vi "ZCAN_InitCAN( CANET ).vi"(0 "设备类型":u32, 5 "device_hande":u32, 7 "CANindex":u32, 9 "ZCAN_InitCAN_setting_CANET":T1, 11 "error in (no error)":errorcluster caption="错误输入（无错误）") -> (8 "can_index_handle":u32, 15 "error out":errorcluster caption="错误输出")   [LabVIEW 2018]
doc: "用于设置CAN通道的初始化参数。\n\n适用的设备：CANET-TCP ,CANET-UDP"
uses:
  zlgcan_demo_CANFDNET_UDP/bin/zlgcan_wrap.dll
  data_type/ZCAN_InitCAN_setting_CANET.ctl
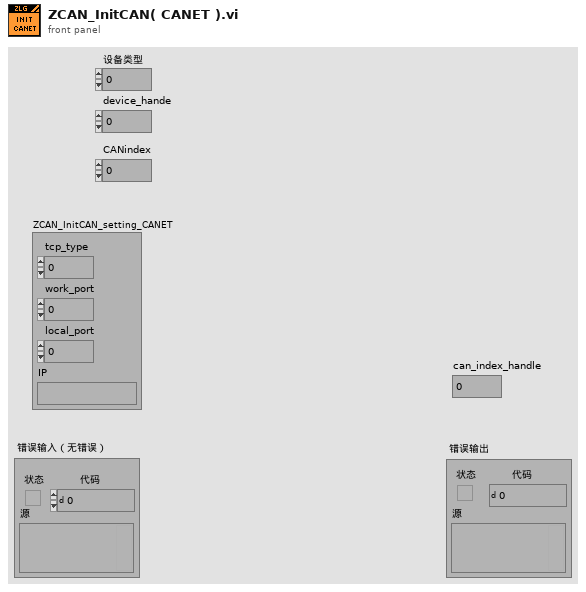
[diagram p1: front panel]
types:
  T1 = typedef "ZCAN_InitCAN_setting_CANET.ctl" = cluster{"tcp_type":u32, "work_port":u32, "local_port":u32, "IP":string}
  T2 = cluster{"can_type":u32, "can_type":u32, "can_type":u32, "can_type":u32, "can_type":u32, "can_type":u32, u8, u8, "pad":u16, "reserved":u32}
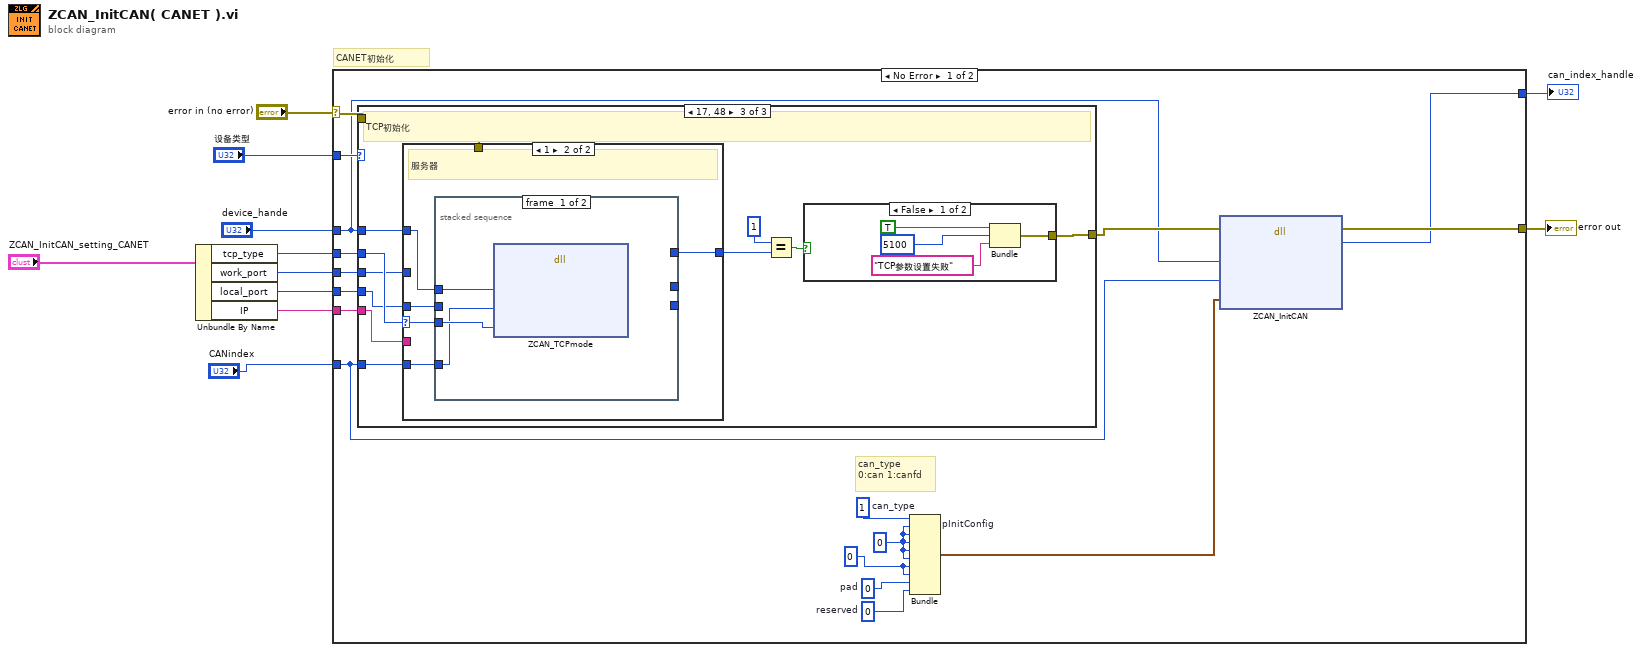
[diagram p0: block diagram]
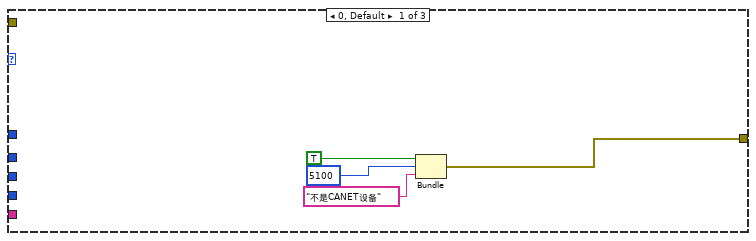
[diagram p2: hidden frame]
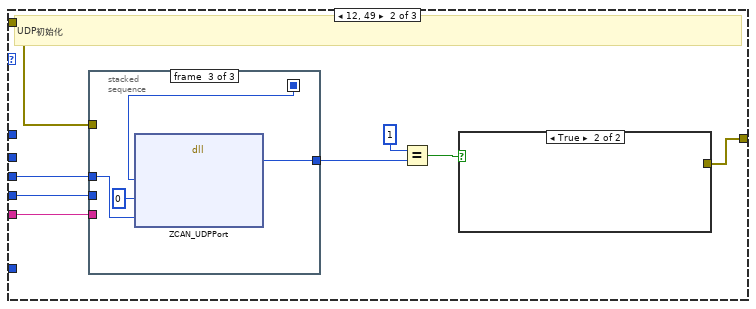
[diagram p3: hidden frame]
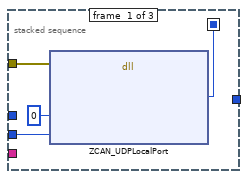
[diagram p4: hidden frame]
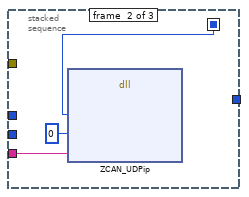
[diagram p5: hidden frame]
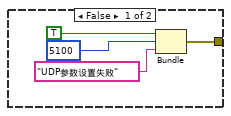
[diagram p6: hidden frame]
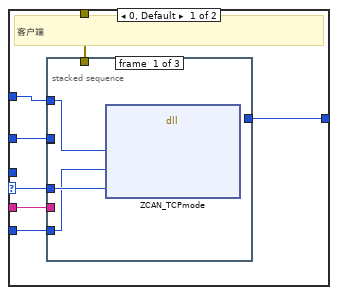
[diagram p7: hidden frame]
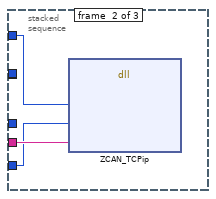
[diagram p8: hidden frame]
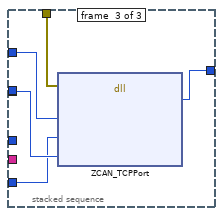
[diagram p9: hidden frame]
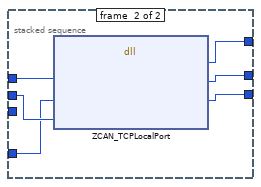
[diagram p10: hidden frame]
diagram:
  # "CANET初始化"
  n1 = Unbundle By Name("ZCAN_InitCAN_setting_CANET") -> ("tcp_type"=w9:u32, "work_port"=w7:u32, "local_port"=w6:u32, "IP"=w8:string)
  n2 = case shown="No Error" "error in (no error)" {
    selector: "error in (no error)" -> [w24 w104]
    tunnel: [w16 w104] -> w4
    tunnel: "设备类型" -> [w23 _]
    tunnel: "device_hande" -> [w14 w103]
    tunnel: w9 -> [w28 _]
    tunnel: w8 -> [w27 _]
    tunnel: w7 -> [w26 _]
    tunnel: w6 -> [w25 _]
    tunnel: [w13 w103] -> w5
    tunnel: "CANindex" -> [w12 _]
    frame No Error {
      w18 = u8 0
      w20 = u32 0  # reserved
      w21 = u16 0  # pad
      w19 = u32 0 ("can_type")
      w22 = u32 1  # can_type
      # "can_type\n0:can 1:canfd"
      n3 = case "条件结构" shown="17, 48" w23 {
        tunnel: [w29 w40 w58] -> w17
        tunnel: w14 -> [_ _ w63]
        tunnel: w28 -> [_ _ w62]
        tunnel: w27 -> [_ w38 w61]
        tunnel: w26 -> [_ w37 w60]
        tunnel: w25 -> [_ w39 w57]
        tunnel: w24 -> [_ w33 w59]
        tunnel: w12 -> [_ _ w56]
        frame 0, Default {
          n4 = Bundle("status"=TRUE, "code"=5100, "消息"="不是CANET设备") -> (w29:cluster{"status":bool, "code":i32, "消息":string})  [unwired: 1 in]
        }
        frame 12, 49 {
          # "UDP初始化"
          n5 = stacked-sequence {
            seq-local: [w41 _ _] -> [_ w45 w48]
            tunnel: w39 -> [w43 _ _]
            tunnel: w38 -> [_ w47 _]
            tunnel: w37 -> [_ _ w51]
            tunnel: [_ _ w49] -> w34
            tunnel: w33 -> [w42 _ _]
            frame #0 {
              n6 = dll-call lib="C:/Users/admin/Desktop/zlgcan_demo_CANFDNET_UDP/bin/zlgcan_wrap.dll" fn="ZCAN_UDPLocalPort"(error in=w42, "can_index"=u32 0, "local_port"=w43) -> ("hDev"=w41:u32)  [unwired: 6 in, 2 out]
            }
            frame #1 {
              n7 = dll-call lib="C:/Users/admin/Desktop/zlgcan_demo_CANFDNET_UDP/bin/zlgcan_wrap.dll" fn="ZCAN_UDPip"("device_handle"=w45, "can_index"=u32 0, "ip"=w47) -> ()  [unwired: 7 in, 2 out]
            }
            frame #2 {
              n8 = dll-call lib="C:/Users/admin/Desktop/zlgcan_demo_CANFDNET_UDP/bin/zlgcan_wrap.dll" fn="ZCAN_UDPPort"("hDev"=w48, "can_index"=u32 0, "work_port"=w51) -> ("return"=w49:u32)  [unwired: 6 in, 2 out]
            }
          }
          n9 = Equal?(x=1, y=w34) -> (x = y?=w35:bool)
          n10 = case shown="True" w35 {
            tunnel: [w52 _] -> w40
            frame False {
              n11 = Bundle("status"=TRUE, "code"=5100, "消息"="UDP参数设置失败") -> (w52:cluster{"status":bool, "code":i32, "消息":string})  [unwired: 1 in]
            }
            frame True {
            }
          }
        }
        frame 17, 48 {
          # "TCP初始化"
          n12 = case shown="1" w62 {
            selector: w62 -> [w73 w89]
            tunnel: [w72 w88] -> w65
            tunnel: w63 -> [w71 w87]
            tunnel: w61 -> [w70 _]
            tunnel: w60 -> [w69 _]
            tunnel: w59 -> [w68 _]
            tunnel: w57 -> [_ w86]
            tunnel: w56 -> [w67 w85]
            frame 0, Default {
              # "客户端"
              n13 = stacked-sequence {
                tunnel: w73 -> [w76 _ _]
                tunnel: [_ _ w84] -> w72
                tunnel: w71 -> [w75 w78 w83]
                tunnel: w70 -> [_ w79 _]
                tunnel: [_ _ w82] -> _
                tunnel: w69 -> [_ _ w82]
                tunnel: w68 -> [_ _ w81]
                tunnel: w67 -> [w74 w77 w80]
                frame #0 {
                  n14 = dll-call lib="C:/Users/admin/Desktop/zlgcan_demo_CANFDNET_UDP/bin/zlgcan_wrap.dll" fn="ZCAN_TCPmode"("hDev"=w75, "can_index"=w74, "tcp_type"=w76) -> ()  [unwired: 7 in, 2 out]
                }
                frame #1 {
                  n15 = dll-call lib="C:/Users/admin/Desktop/zlgcan_demo_CANFDNET_UDP/bin/zlgcan_wrap.dll" fn="ZCAN_TCPip"("device_handle"=w78, "can_index"=w77, "ip"=w79) -> ()  [unwired: 7 in, 2 out]
                }
                frame #2 {
                  n16 = dll-call lib="C:/Users/admin/Desktop/zlgcan_demo_CANFDNET_UDP/bin/zlgcan_wrap.dll" fn="ZCAN_TCPPort"(error in=w81, "hDev"=w83, "can_index"=w80, "work_port"=w82) -> ("return"=w84:u32)  [unwired: 5 in, 2 out]
                }
              }
            }
            frame 1 {
              # "服务器"
              n17 = stacked-sequence {
                tunnel: w89 -> [w92 _]
                tunnel: [_ w98] -> w88
                tunnel: [_ w97] -> _
                tunnel: [_ w96] -> _
                tunnel: w87 -> [w91 w94]
                tunnel: w86 -> [_ w95]
                tunnel: w85 -> [w90 w93]
                frame #0 {
                  n18 = dll-call lib="C:/Users/admin/Desktop/zlgcan_demo_CANFDNET_UDP/bin/zlgcan_wrap.dll" fn="ZCAN_TCPmode"("hDev"=w91, "can_index"=w90, "tcp_type"=w92) -> ()  [unwired: 7 in, 2 out]
                }
                frame #1 {
                  n19 = dll-call lib="C:/Users/admin/Desktop/zlgcan_demo_CANFDNET_UDP/bin/zlgcan_wrap.dll" fn="ZCAN_TCPLocalPort"("device_handle"=w94, "can_index"=w93, "local_port"=w95) -> ("return"=w98:u32, "device_handle"=w97:u32, "can_index"=w96:u32)  [unwired: 4 in, 2 out]
                }
              }
            }
          }
          n20 = Equal?(x=1, y=w65) -> (x = y?=w64:bool)
          n21 = case shown="False" w64 {
            tunnel: [w99 _] -> w58
            frame False {
              n22 = Bundle("status"=TRUE, "code"=5100, "消息"="TCP参数设置失败") -> (w99:cluster{"status":bool, "code":i32, "消息":string})  [unwired: 1 in]
            }
            frame True {
            }
          }
        }
      }
      n23 = Bundle "pInitConfig"("can_type"=w22, "can_type"=w19, "can_type"=w19, "can_type"=w19, "can_type"=w19, "can_type"=w19, w18, w18, "pad"=w21, "reserved"=w20) -> (w15:T2)  [unwired: 1 in]
      n24 = dll-call lib="C:/Users/admin/Desktop/zlgcan_demo_CANFDNET_UDP/bin/zlgcan_wrap.dll" fn="ZCAN_InitCAN"(error in=w17, "device_handle"=w14, "can_index"=w12, "pInitConfig"=w15) -> (error out=w16:errorcluster, "can_handle"=w13:u32)  [unwired: 5 in, 1 out]
    }
    frame Error {
    }
  }
  "error out" <- w4
  "can_index_handle" <- w5
